vi "rotate.vi"(0 "Angle":dbl, 1 "Rate":dbl=-4.0) -> (2 "finished?":bool, 3 "left speed":dbl, 4 "right speed":dbl)   [LabVIEW 2011]
doc: "Rotates the robot for a certain number of degrees at a certain rate."
uses:
  subStates.ctl
  <vilib>/addons/control/pid/pid.llb/PID Control Input Filter (DBL).vi
  <vilib>/addons/control/pid/pid.llb/PID (DBL).vi
  <vilib>/addons/control/pid/NI_PID_pid.lvlib
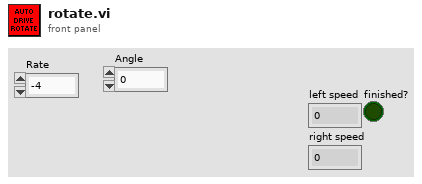
[diagram p1: front panel]
types:
  T1 = cluster{"proportional gain (Kc)":dbl, "integral time (Ti, min)":dbl, "derivative time (Td, min)":dbl}
  T2 = typedef "subStates.ctl" = enum16{"null", "wait", "driver control", "auto", "manual override", "autoDrive", "hold position", "rotate", "end"}
  T3 = typedef "WPI_EncoderDevRef.ctl" = cluster{"DevStatus":errorcluster, "EncoderIndex":T4, "CounterIndex":T5, "DistancePerCount":dbl, "Decoding Type":T6}
  T4 = typedef "FPGA_EncoderIdx.ctl" = enum8{"Enc 0", "Enc 1", "Enc 2", "Enc 3", "Invalid"}
  T5 = typedef "FPGA_CounterCtrSystemIndex.ctl" = enum8{"Ctr 0", "Ctr 1", "Ctr 2", "Ctr 3", "Ctr 4", "Ctr 5", "Ctr 6", "Ctr 7", "Invalid"}
  T6 = typedef "WPI_EncoderType.ctl" = enum16{"1x", "2x", "4x"}
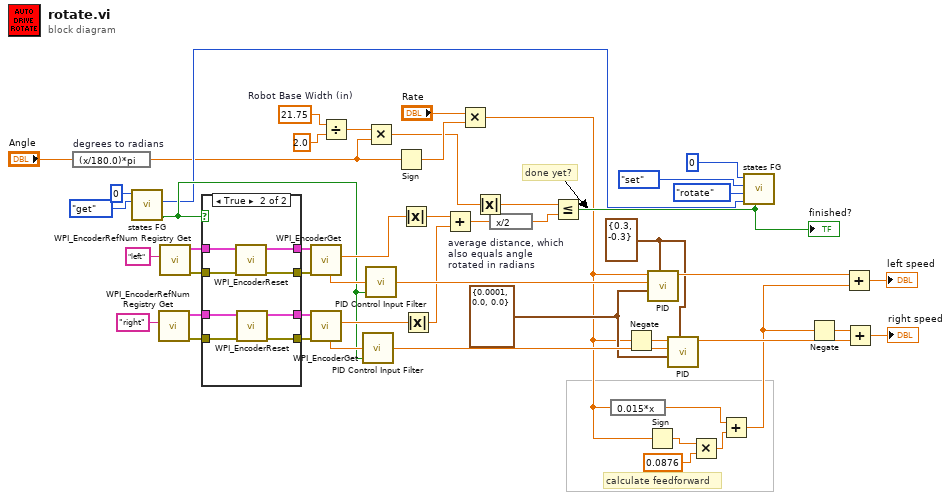
[diagram p0: block diagram]
diagram:
  w18 = T1 {"proportional gain (Kc)"=0.0001, "integral time (Ti, min)"=0.0, "derivative time (Td, min)"=0.0} ("PID gains")
  w46 = cluster{"output high":dbl, "output low":dbl} {"output high"=0.3, "output low"=-0.3} ("output range")
  w50 = 21.75  # Robot Base Width (in)
  # "calculate feedforward"
  # "done yet?"
  n1 = expression code="(x/180.0)*pi" "degrees to radians"("Angle") -> (w2:dbl)
  n2 = call "states FG.vi"("menu (get)"=enum16{"set", "get"}."get", "Loop ID"=0) -> ("first call?"=w19:bool, "state # out"=w4:i32)  [unwired: 6 in, 2 out]
  n3 = call <vilib>:"WPI_EncoderRefNum Registry Get.vi"("refnum name"="right") -> ("error out"=w30:errorcluster, "EncoderDevRef"=w31:T3)  [unwired: 9 in]
  n4 = call <vilib>:"WPI_EncoderRefNum Registry Get.vi"("refnum name"="left") -> ("error out"=w32:errorcluster, "EncoderDevRef"=w33:T3)  [unwired: 9 in]
  n5 = case shown="True" w19 {
    tunnel: w33 -> [w55 w61]
    tunnel: w32 -> [w54 w63]
    tunnel: w31 -> [w53 w58]
    tunnel: w30 -> [w52 w59]
    tunnel: [w54 w62] -> w29
    tunnel: [w55 w60] -> w28
    tunnel: [w53 w57] -> w27
    tunnel: [w52 w56] -> w26
    frame False {
    }
    frame True {
      n6 = call <vilib>:"WPI_EncoderReset.vi"("error in (no error)"=w63, "EncoderDevRef"=w61) -> ("error out"=w62:errorcluster, "EncoderDevRef"=w60:T3)  [unwired: 8 in]
      n7 = call <vilib>:"WPI_EncoderReset.vi"("error in (no error)"=w59, "EncoderDevRef"=w58) -> ("error out"=w56:errorcluster, "EncoderDevRef"=w57:T3)  [unwired: 8 in]
    }
  }
  n8 = call <vilib>:"WPI_EncoderGet.vi"("error in (no error)"=w29, "EncoderDevRef"=w28) -> ("Distance"=w25:dbl, "Rate"=w40:dbl)  [unwired: 4 in, 4 out]
  n9 = call <vilib>:"WPI_EncoderGet.vi"("error in (no error)"=w26, "EncoderDevRef"=w27) -> ("Distance"=w24:dbl, "Rate"=w39:dbl)  [unwired: 4 in, 4 out]
  n10 = Divide(x=w50, y=2.0) -> (x/y=w49:dbl)
  n11 = call-poly <vilib>:"PID Control Input Filter.vi"("reinitialize? (F)"=w19, "input"=w39) -> ("output"=w20:dbl)  [unwired: 3 in]
  n12 = Multiply(x=w49, y=w2) -> (x*y=w15:dbl)
  n13 = call-poly <vilib>:"PID Control Input Filter.vi"("reinitialize? (F)"=w19, "input"=w40) -> ("output"=w21:dbl)  [unwired: 3 in]
  n14 = Sign(1:w2) -> (0:w16:dbl)
  n15 = Absolute Value(x=w25) -> (abs(x)=w14:dbl)
  n16 = Absolute Value(x=w24) -> (abs(x)=w13:dbl)
  n17 = Add(x=w14, y=w13) -> (x+y=w38:dbl)
  n18 = Multiply(x="Rate", y=w16) -> (x*y=w9:dbl)
  n19 = Absolute Value(x=w15) -> (abs(x)=w1:dbl)
  n20 = expression code="x/2" "average distance, which also equals angle rotated in radians"(w38) -> (w37:dbl)
  n21 = Less Or Equal?(x=w1, y=w37) -> (x <= y?=w36:bool)
  "finished?" <- w36
  n22 = expression code="0.015*x"(w9) -> (w7:dbl)
  n23 = Negate(x=w9) -> (-x=w12:dbl)
  n24 = Sign(1:w9) -> (0:w11:dbl)
  n25 = call-poly <vilib>:"PID.vi"("output range"=w46, "PID gains"=w18, "process variable"=w21, "setpoint"=w9) -> ("output"=w47:dbl)  [unwired: 6 in, 1 out]
  n26 = call-poly <vilib>:"PID.vi"("output range"=w46, "PID gains"=w18, "process variable"=w20, "setpoint"=w12) -> ("output"=w48:dbl)  [unwired: 6 in, 1 out]
  n27 = Multiply(x=w11, y=0.0876) -> (x*y=w8:dbl)
  n28 = Add(x=w7, y=w8) -> (x+y=w5:dbl)
  n29 = call "states FG.vi"("exit in"=w36, "state # in"=w4, "subState in"=subStates."rotate", "menu (get)"=enum16{"set", "get"}."set", "Loop ID"=0) -> ()  [unwired: 3 in, 4 out]
  n30 = Negate(x=w5) -> (-x=w6:dbl)
  n31 = Add(x=w47, y=w5) -> (x+y=→"left speed":dbl)
  n32 = Add(x=w6, y=w48) -> (x+y=→"right speed":dbl)
